vi "ComConnect.vi"(0 "Action":enum16{"Open", "Get ID", "Close"}(ring)) -> (1 "ConnectID":u32, 2 "err":bool, 3 "Err Msg":string)   [LabVIEW 2011]
uses:
  Globals/CTCGlbs.vi
  Windows/System32/Ctccom32v2.dll
  Ctccom32v2.dll
panel:
  in  "BaudRate":u32=9600
  in  "Type":T1(ring)=enum."Ethernet"
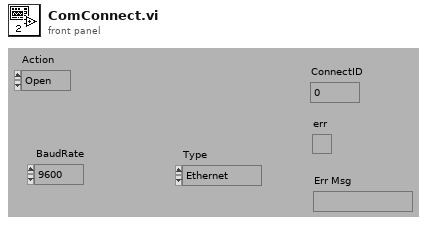
[diagram p1: front panel]
types:
  T1 = enum16{"No Connection", "Serial", "Ethernet", "Web"}
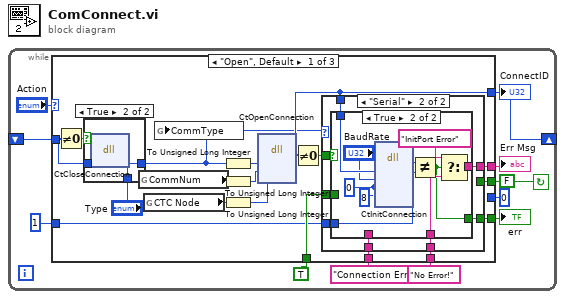
[diagram p0: block diagram]
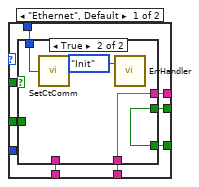
[diagram p2: hidden frame]
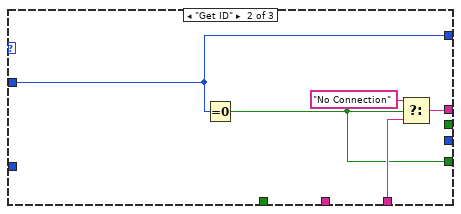
[diagram p6: hidden frame]
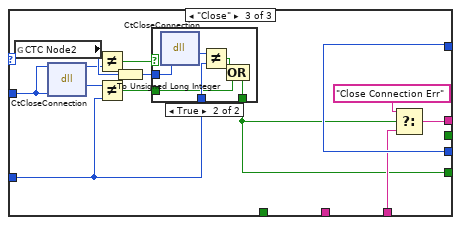
[diagram p7: hidden frame]
diagram:
  n1 = while {
    shift-left: _ -> [w10]
    shift-right: [w7] -> _
    stop <- w1 continue-if-true
    w1 = FALSE
    n2 = case shown="\"Open\", Default" "Action" {
      tunnel: w10 -> [w28 w71 w74]
      tunnel: [w27 w71 w83] -> w7
      tunnel: u32 1 -> [w17 _ w78]
      tunnel: u32 0 -> [_ _ w83]
      tunnel: "No Error!" -> [w26 w70 w81]
      tunnel: [w25 w69 w80] -> w5
      tunnel: "Connection Err" -> [w24 _ _]
      tunnel: [w22 w67 w76] -> w3
      tunnel: TRUE -> [w23 _ _]
      tunnel: w1 -> [w21 _ _]
      frame "Open", Default {
        n3 = Not Equal To 0?(x=w28) -> (x != 0?=w29:bool)
        n4 = case shown="True" w29 {
          tunnel: w28 -> [_ w66]
          tunnel: "Type" -> [w64 w65]
          tunnel: [w64 w65] -> w15
          frame False {
          }
          frame True {
            n5 = dll-call lib="C:/WINNT/system32/CtcEmcorev2.dll" fn="CtCloseConnection"("ConnectID"=w66) -> ()  [unwired: 5 in, 2 out]
          }
        }
        n6 = global read "CTCGlbs.vi" "CommNum"() -> (w18:i16)
        n7 = global read "CTCGlbs.vi" "CTC Node"() -> (w20:i16)
        n8 = global write "CTCGlbs.vi" "CommType"(w15) -> ()
        n9 = To Unsigned Long Integer(number=w15) -> (unsigned 32bit integer=w14:u32)
        n10 = To Unsigned Long Integer(number=w18) -> (unsigned 32bit integer=w12:u32)
        n11 = To Unsigned Long Integer(number=w20) -> (unsigned 32bit integer=w13:u32)
        n12 = dll-call lib="C:/Users/MOCVD/Downloads/Labview/Ctccom32v2/Ctccom32v2.dll" fn="CtOpenConnection"("ConnectType"=w14, "LocalAddress"=w12, "RemotAddress"=w13) -> (w27:u32)  [unwired: 6 in, 2 out]
        n13 = Not Equal To 0?(x=w27) -> (x != 0?=w19:bool)
        n14 = case shown="\"Serial\"" w15 {
          tunnel: w27 -> [w30 w51]
          tunnel: w19 -> [w37 w50]
          tunnel: w17 -> [_ w49]
          tunnel: w26 -> [w36 w48]
          tunnel: [w35 w47] -> w25
          tunnel: w24 -> [w34 w46]
          tunnel: w21 -> [w33 _]
          tunnel: [w32 w45] -> w22
          tunnel: w23 -> [w31 w44]
          frame "Ethernet", Default {
            n15 = case shown="True" w37 {
              tunnel: [w39 w42] -> w35
              tunnel: w36 -> [_ w42]
              tunnel: w34 -> [w39 _]
              tunnel: w33 -> [_ w41]
              tunnel: [w38 w41] -> w32
              tunnel: w31 -> [w38 _]
              tunnel: w30 -> [_ w40]
              frame False {
              }
              frame True {
                n16 = call "SetCtComm.vi"("ConnectID"=w40) -> ()  [unwired: 1 in]
                n17 = call "ErrHandler.vi"("Action"=enum16{"Init", "Process"}."Init") -> ()  [unwired: 1 in, 1 out]
              }
            }
          }
          frame "Serial" {
            n18 = case shown="True" w50 {
              tunnel: w51 -> [_ w63]
              tunnel: w49 -> [_ w58]
              tunnel: w48 -> [_ w56]
              tunnel: [w53 w55] -> w47
              tunnel: w46 -> [w53 _]
              tunnel: [w52 w54] -> w45
              tunnel: w44 -> [w52 _]
              frame False {
              }
              frame True {
                w61 = u8 0
                n19 = dll-call lib="C:/WINNT/system32/CtcEmcorev2.dll" fn="CtInitConnection"("ConnectID"=w63, "BaudRate"="BaudRate", "Parity"=w61, "DataBits"=u8 8, "StopBits"=w61) -> (w59:u32)  [unwired: 8 in, 2 out]
                n20 = Not Equal?(x=w59, y=w58) -> (x != y?=w54:bool)
                n21 = Select(t="InitPort Error", s=w54, f=w56) -> (s? t:f=w55:string)
              }
            }
          }
        }
      }
      frame "Get ID" {
        n22 = Equal To 0?(x=w71) -> (x = 0?=w67:bool)
        n23 = Select(t="No Connection", s=w67, f=w70) -> (s? t:f=w69:string)
      }
      frame "Close" {
        n24 = global read "CTCGlbs.vi" "CTC Node2"() -> (w75:i16)
        n25 = dll-call lib="C:/WINNT/system32/CtcEmcorev2.dll" fn="CtCloseConnection"("ConnectID"=w74) -> (w73:u32)  [unwired: 4 in, 2 out]
        n26 = Not Equal?(x=w75, y=w74) -> (x != y?=w79:bool)
        n27 = Not Equal?(x=w73, y=w78) -> (x != y?=w77:bool)
        n28 = To Unsigned Long Integer(number=w75) -> (unsigned 32bit integer=w72:u32)
        n29 = case shown="True" w79 {
          tunnel: w78 -> [_ w90]
          tunnel: w77 -> [w84 w88]
          tunnel: [w84 w87] -> w76
          tunnel: w72 -> [_ w85]
          frame False {
          }
          frame True {
            n30 = dll-call lib="C:/WINNT/system32/CtcEmcorev2.dll" fn="CtCloseConnection"("ConnectID"=w85) -> (w86:u32)  [unwired: 4 in, 2 out]
            n31 = Not Equal?(x=w86, y=w90) -> (x != y?=w89:bool)
            n32 = Compound Arithmetic op=OR(w89, w88) -> (w87:bool)
          }
        }
        n33 = Select(t="Close Connection Err", s=w76, f=w81) -> (s? t:f=w80:string)
      }
    }
    "Err Msg" <- w5
    "ConnectID" <- w7
    "err" <- w3
  }
